vi "Set bottom frame colors.vi"(4 "Bolts":u32(colorbox), 6 "Supports":u32(colorbox), 8 "error in (no error)":errorcluster, 9 "Frame connectors":u32(colorbox), 10 "Metal frame":u32(colorbox), 11 "Detector ref in":refnum<vi>) -> (0 "error out":errorcluster, 3 "Detector ref out":refnum<vi>)   [LabVIEW 2016]
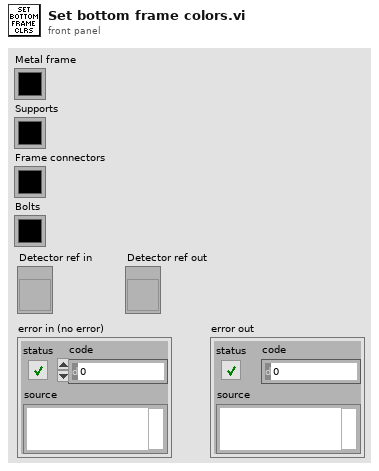
[diagram p1: front panel]
types:
  T1 = typedef "LVRGBAColorTypeDef.ctl" = cluster{"Red":sgl, "Green":sgl, "Blue":sgl, "Alpha":sgl}
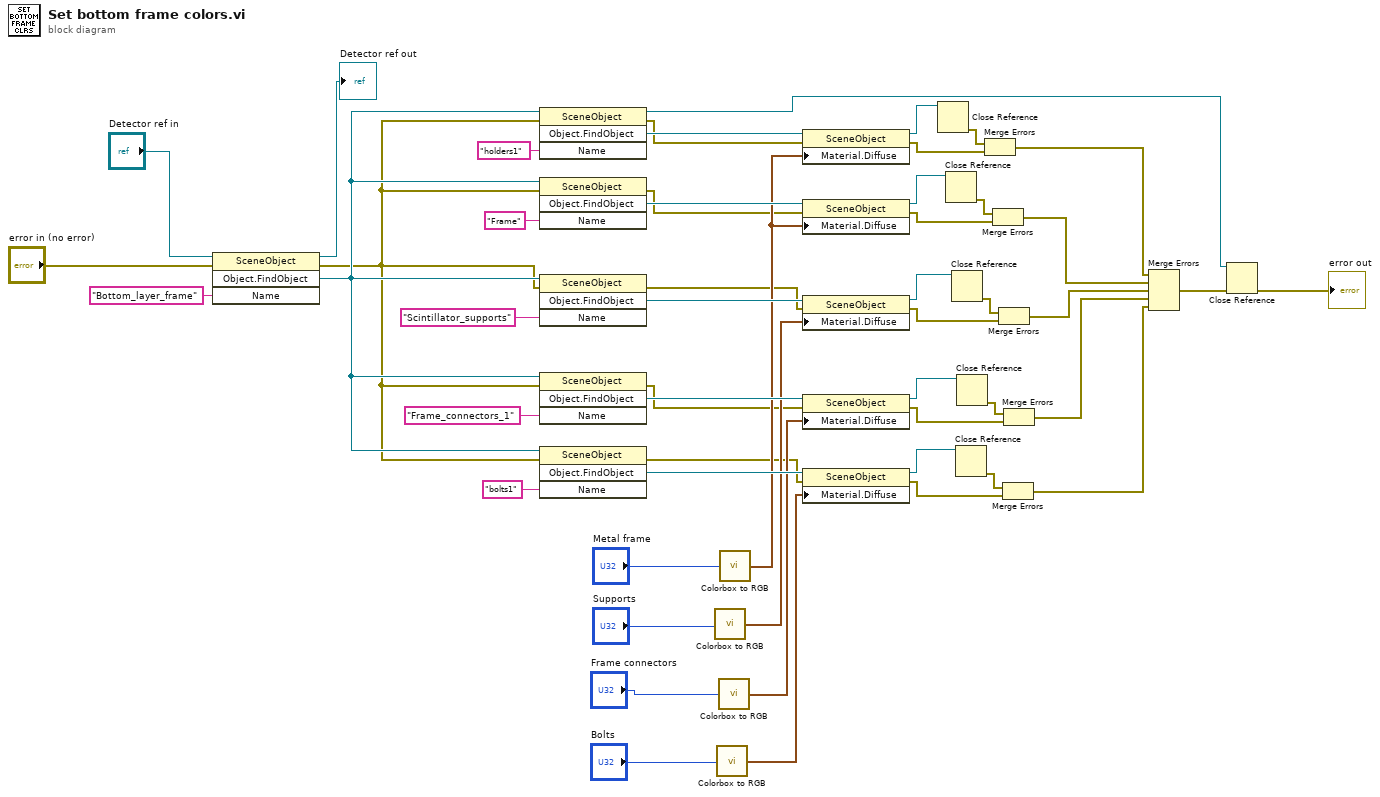
[diagram p0: block diagram]
diagram:
  n1 = invoke class="SceneObject" method="Object.FindObject"(reference="Detector ref in", error in="error in (no error)", "Name"="Bottom_layer_frame") -> (reference out=→"Detector ref out":refnum<vi>, error out=w29:errorcluster, "FindObject"=w51:refnum<vi>)  [unwired: 1 in, 1 out]
  n2 = invoke class="SceneObject" method="Object.FindObject"(reference=w51, error in=w29, "Name"="holders1") -> (reference out=w1:refnum<vi>, error out=w4:errorcluster, "FindObject"=w45:refnum<vi>)  [unwired: 1 in, 1 out]
  n3 = invoke class="SceneObject" method="Object.FindObject"(reference=w51, error in=w29, "Name"="Frame") -> (error out=w8:errorcluster, "FindObject"=w46:refnum<vi>)  [unwired: 1 in, 2 out]
  n4 = invoke class="SceneObject" method="Object.FindObject"(reference=w51, error in=w29, "Name"="Scintillator_supports") -> (error out=w7:errorcluster, "FindObject"=w42:refnum<vi>)  [unwired: 1 in, 2 out]
  n5 = invoke class="SceneObject" method="Object.FindObject"(reference=w51, error in=w29, "Name"="Frame_connectors_1") -> (error out=w6:errorcluster, "FindObject"=w49:refnum<vi>)  [unwired: 1 in, 2 out]
  n6 = invoke class="SceneObject" method="Object.FindObject"(reference=w51, error in=w29, "Name"="bolts1") -> (error out=w5:errorcluster, "FindObject"=w52:refnum<vi>)  [unwired: 1 in, 2 out]
  n7 = call "Colorbox to RGB.vi"("Color"="Supports") -> ("Material"=w38:T1)
  n8 = call "Colorbox to RGB.vi"("Color"="Bolts") -> ("Material"=w36:T1)
  n9 = call "Colorbox to RGB.vi"("Color"="Frame connectors") -> ("Material"=w37:T1)
  n10 = call "Colorbox to RGB.vi"("Color"="Metal frame") -> ("Material"=w39:T1)
  n11 = property class="SceneObject"(reference=w45, error in=w4, "Material.Diffuse"=w39) -> (reference out=w23:refnum<vi>, error out=w22:errorcluster)
  n12 = property class="SceneObject"(reference=w46, error in=w8, "Material.Diffuse"=w39) -> (reference out=w21:refnum<vi>, error out=w20:errorcluster)
  n13 = property class="SceneObject"(reference=w42, error in=w7, "Material.Diffuse"=w38) -> (reference out=w19:refnum<vi>, error out=w18:errorcluster)
  n14 = property class="SceneObject"(reference=w49, error in=w6, "Material.Diffuse"=w37) -> (reference out=w17:refnum<vi>, error out=w16:errorcluster)
  n15 = property class="SceneObject"(reference=w52, error in=w5, "Material.Diffuse"=w36) -> (reference out=w15:refnum<vi>, error out=w14:errorcluster)
  n16 = Close Reference(reference=w23) -> (error out=w28:errorcluster)  [unwired: 1 in]
  n17 = Close Reference(reference=w21) -> (error out=w27:errorcluster)  [unwired: 1 in]
  n18 = Close Reference(reference=w19) -> (error out=w26:errorcluster)  [unwired: 1 in]
  n19 = Close Reference(reference=w15) -> (error out=w24:errorcluster)  [unwired: 1 in]
  n20 = Close Reference(reference=w17) -> (error out=w25:errorcluster)  [unwired: 1 in]
  n21 = Merge Errors(w28, w22) -> (w13:errorcluster)
  n22 = Merge Errors(w27, w20) -> (w12:errorcluster)
  n23 = Merge Errors(w26, w18) -> (w11:errorcluster)
  n24 = Merge Errors(w24, w14) -> (w9:errorcluster)
  n25 = Merge Errors(w25, w16) -> (w10:errorcluster)
  n26 = Merge Errors(w13, w12, w11, w10, w9) -> (w3:errorcluster)
  n27 = Close Reference(reference=w1, error in (no error)=w3) -> (error out=→"error out":errorcluster)
